vi "sv_Equivalent Continuous Level with IC_octave.vi"(2 "init/cont (init:F)":bool, 3 "initial internal state":cluster{"squared sum":dbl, "size":dbl} {"size" format="%.2f"; "squared sum" format="%.2f"}, 4 "scaled signal [EU]":dbl[](array[numeric]) format="%.2f") -> (0 "final internal state":cluster{"squared sum":dbl, "size":dbl} {"size" format="%.2f"; "squared sum" format="%.2f"}, 1 "equivalent continuous level [EU^2 rms]":dbl format="%.2f")   [LabVIEW 2017]
doc: "Computes the equivalent continuous level of the input signal.\nThe initial internal state and final internal state keep track of the internal state of the averaging process to ensure continuous operation if you use continuous mode."
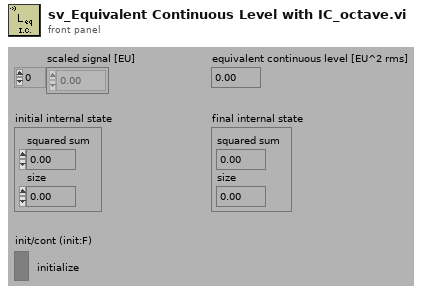
[diagram p1: front panel]
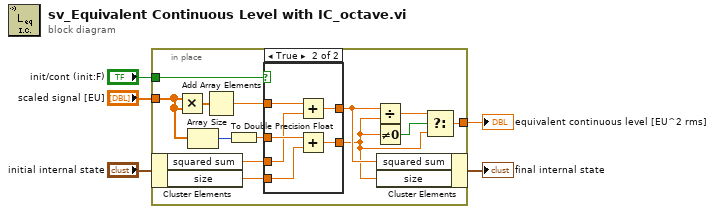
[diagram p0: block diagram]
diagram:
  n1 = in-place {
    in-place-border: "init/cont (init:F)" -> [w17]
    in-place-border: "scaled signal [EU]" -> [w15]
    in-place-border: [w10] -> w3
    n2 = in-place-cluster #1("initial internal state") -> ("squared sum"=w9:dbl, "size"=w8:dbl)
    n3 = Multiply(x=w15, y=w15) -> (x*y=w13:dbl[])
    n4 = Array Size(array=w15) -> (size(s)=w18:i32)
    n5 = Add Array Elements(numeric array=w13) -> (sum=w14:dbl)
    n6 = To Double Precision Float(number=w18) -> (double precision float=w16:dbl)
    n7 = case shown="True" w17 {
      tunnel: w14 -> [w20 w23]
      tunnel: w16 -> [w19 w26]
      tunnel: [w19 w25] -> w6
      tunnel: [w20 w24] -> w7
      tunnel: w9 -> [_ w22]
      tunnel: w8 -> [_ w21]
      frame False {
      }
      frame True {
        n8 = Add(x=w23, y=w22) -> (x+y=w24:dbl)
        n9 = Add(x=w26, y=w21) -> (x+y=w25:dbl)
      }
    }
    n10 = Divide(x=w7, y=w6) -> (x/y=w11:dbl)
    n11 = Not Equal To 0?(x=w6) -> (x != 0?=w12:bool)
    n12 = in-place-cluster #1("squared sum"=w7, "size"=w6) -> (→"final internal state":cluster{"squared sum":dbl, "size":dbl})
    n13 = Select(t=w11, s=w12, f=w6) -> (s? t:f=w10:dbl)
  }
  "equivalent continuous level [EU^2 rms]" <- w3
